vi "Set Analog In Trigger.vi"(8 "error in (no error)":errorcluster, 9 "timeout":dbl, 10 "trigsrc":T1, 11 "hdwf":i32) -> (0 "error out":errorcluster, 3 "hdwf out":i32)   [LabVIEW 2012, in "AnalogDiscSDKLv.lvlib"]
doc: "extern \"C\" __declspec(dllexport) int Set_AnalogIn_Trigger(HDWF hdwf, TRIGSRC trigsrc, double timeout);"
uses:
  <instrlib>/AnalogDiscSDKLv/AnalogDiscSDKLv.lvlib
  <instrlib>/AnalogDiscSDKLv/VIs/DWF_TrigSrc.ctl
  <instrlib>/AnalogDiscSDKLv/AnalogDiscSDKLv.dll
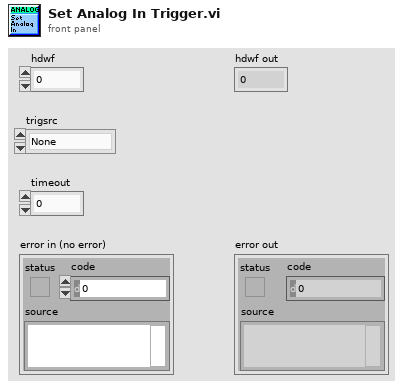
[diagram p1: front panel]
types:
  T1 = typedef "DWF_TrigSrc.ctl" = enum16{"None", "PC", "DetectorAnalogIn", "DetectorDigitalIn", "AnalogIn", "DigitalIn", "DigitalOut", "AnalogOut1", "AnalogOut2", "AnalogOut3", "AnalogOut4", "External1", "External2", "External3", "External4"}
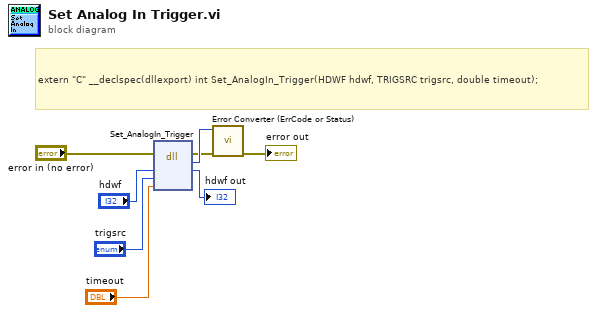
[diagram p0: block diagram]
diagram:
  # "extern \"C\" __declspec(dllexport) int Set_AnalogIn_Trigger(HDWF hdwf, TRIGSRC trigsrc, double timeout);"
  n1 = dll-call lib="C:/Program Files (x86)/National Instruments/LabVIEW 2012/instr.lib/AnalogDiscSDKLv/AnalogDiscSDKLv.*" fn="Set_AnalogIn_Trigger"(error in="error in (no error)", "hdwf"="hdwf", "trigsrc"="trigsrc", "timeout"="timeout") -> (error out=w2:errorcluster, "return type"=w3:i32, "hdwf"=→"hdwf out":i32)  [unwired: 4 in, 1 out]
  n2 = call <instrlib>:"Error Converter (ErrCode or Status).vi"("error in (no error)"=w2, "error code"=w3) -> ("error out"=→"error out":errorcluster)  [unwired: 9 in]
